vi "Schedule Packet Generation Based on Timestamps.vi"(0 "tagged llp packet":T1, 1 "reset":bool, 2 "generation counter":T10, 5 "start trigger":bool, 7 "stop trigger":bool, 9 "tagged llp packet valid":bool, 11 "configuration":T11, 12 "ready to generate packet":bool) -> (3 "in reset":bool, 4 "packet timing error":bool, 6 "packet timing error (cycles)":u64, 8 "number of buffered llp timestamps":u32, 10 "generate packet":bool, 14 "ready for tagged llp packet":bool)   [LabVIEW 2020, in "GettingStarted_Gen_148X_FPGA.lvlib"]
uses:
  GettingStarted_Gen_148X_FPGA.lvlib
  Types/Serial Output Channel Datapath Configuration.ctl
  <instrlib>/FlexRIO/CSI-2/v2/FPGA/Types/Timestamp Counter Value.ctl
  <instrlib>/FlexRIO/CSI-2/v2/FPGA/Types/Tagged LLP Packet.ctl
  <instrlib>/FlexRIO/CSI-2/v2/FPGA/Types/FPGA LLP Packet Tag.ctl
  <instrlib>/FlexRIO/CSI-2/v2/FPGA/Types/FPGA LLP Packet Timestamp.ctl
  <instrlib>/FlexRIO/CSI-2/v2/FPGA/Types/Timestamp ID.ctl
  <instrlib>/FlexRIO/CSI-2/v2/FPGA/Types/FPGA LLP Packet Size.ctl
  <instrlib>/FlexRIO/CSI-2/v2/FPGA/Types/LLP Packet.ctl
  <instrlib>/FlexRIO/CSI-2/v2/FPGA/Types/LLP Packet Header.ctl
  <instrlib>/FlexRIO/CSI-2/v2/FPGA/Types/LLP Packet Payload.ctl
  <instrlib>/FlexRIO/CSI-2/v2/FPGA/Types/LLP Packet Footer.ctl
  <instrlib>/FlexRIO/CSI-2/v2/FPGA/NI CSI-2 API FPGA v2.lvlib
  <instrlib>/_niInstr/Basic Elements/v1/FPGA/niInstr Basic Elements v1 FPGA.lvlib
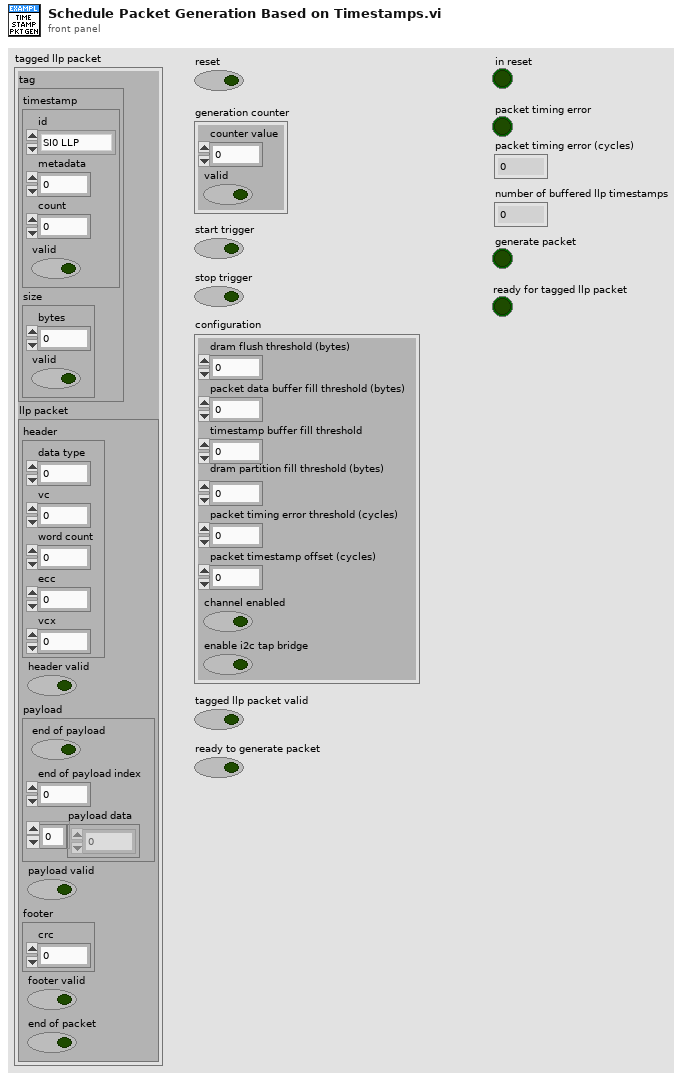
[diagram p1: front panel]
types:
  T1 = typedef "NI CSI-2 API FPGA v2.lvlib/Tagged LLP Packet.ctl" = cluster{"tag":T2, "llp packet":T6}
  T2 = typedef "NI CSI-2 API FPGA v2.lvlib/FPGA LLP Packet Tag.ctl" = cluster{"timestamp":T3, "size":T5}
  T3 = typedef "NI CSI-2 API FPGA v2.lvlib/FPGA LLP Packet Timestamp.ctl" = cluster{"valid":bool, "count":fxp<+,50,50>, "id":T4, "metadata":u8}
  T4 = typedef "NI CSI-2 API FPGA v2.lvlib/Timestamp ID.ctl" = enum8{"SI0 LLP", "SI1 LLP", "SI2 LLP", "SI3 LLP", "SI4 LLP", "SI5 LLP", "SI6 LLP", "SI7 LLP", "SO0 LLP", "SO1 LLP", "SO2 LLP", "SO3 LLP", "SO4 LLP", "SO5 LLP", "SO6 LLP", "SO7 LLP", "Ser0 GPIO Bank", "Ser1 GPIO Bank", "Ser2 GPIO Bank", "Ser3 GPIO Bank", "Ser4 GPIO Bank", "Ser5 GPIO Bank", "Ser6 GPIO Bank", "Ser7 GPIO Bank", "Des0 GPIO Bank", "Des1 GPIO Bank", "Des2 GPIO Bank", "Des3 GPIO Bank", "Des4 GPIO Bank", "Des5 GPIO Bank", "Des6 GPIO Bank", "Des7 GPIO Bank", "User0", "User1", "User2", "User3", "User4", "User5", "User6", "User7", "User8", "User9", "User10", "User11", "User12", "User13", "User14", "User15", "User16", "User17", "User18", "User19", "User20", "User21", "User22", "User23", "User24", "User25", "User26", "User27", "User28", "User29", "User30", "User31"}
  T5 = typedef "NI CSI-2 API FPGA v2.lvlib/FPGA LLP Packet Size.ctl" = cluster{"bytes":fxp<+,17,17>, "valid":bool}
  T6 = typedef "NI CSI-2 API FPGA v2.lvlib/LLP Packet.ctl" = cluster{"header":T7, "header valid":bool, "payload":T8, "payload valid":bool, "footer":T9, "footer valid":bool, "end of packet":bool}
  T7 = typedef "NI CSI-2 API FPGA v2.lvlib/LLP Packet Header.ctl" = cluster{"word count":u16, "ecc":fxp<+,6,6>, "vcx":fxp<+,2,2>, "data type":fxp<+,6,6>, "vc":fxp<+,2,2>}
  T8 = typedef "NI CSI-2 API FPGA v2.lvlib/LLP Packet Payload.ctl" = cluster{"end of payload":bool, "end of payload index":fxp<+,3,3>, "payload data":u8[]}
  T9 = typedef "NI CSI-2 API FPGA v2.lvlib/LLP Packet Footer.ctl" = cluster{"crc":u16}
  T10 = typedef "NI CSI-2 API FPGA v2.lvlib/Timestamp Counter Value.ctl" = cluster{"counter value":u64, "valid":bool}
  T11 = typedef "GettingStarted_Gen_148X_FPGA.lvlib/Serial Output Channel Datapath Configuration.ctl" = cluster{"dram flush threshold (bytes)":u64, "packet data buffer fill threshold (bytes)":u64, "timestamp buffer fill threshold":u32, "packet timing error threshold (cycles)":u64, "channel enabled":bool, "dram partition fill threshold (bytes)":u64, "enable i2c tap bridge":bool, "packet timestamp offset (cycles)":i64}
  T12 = typedef "NI CSI-2 API FPGA v2.lvlib/Raw Timestamp.ctl" = cluster{"timestamp":u64, "valid":bool}
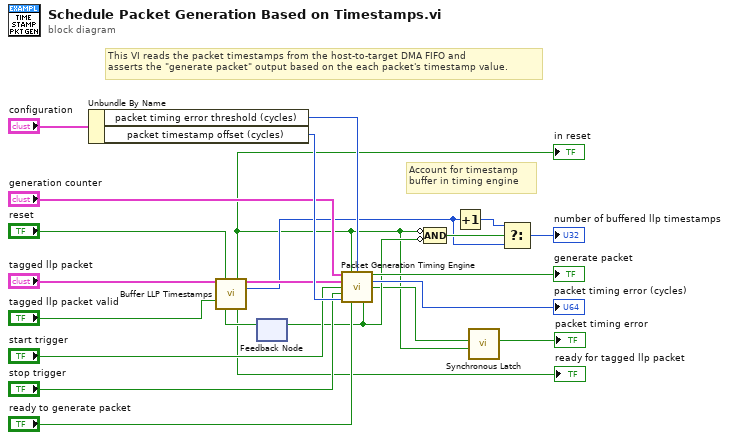
[diagram p0: block diagram]
diagram:
  # "Account for timestamp \nbuffer in timing engine"
  # "This VI reads the packet timestamps from the host-to-target DMA FIFO and \nasserts the \"generate packet\" output based on the each packet's timestamp value."
  n1 = Unbundle By Name("configuration") -> ("packet timing error threshold (cycles)"=w20:u64, "packet timestamp offset (cycles)"=w23:i64)
  n2 = feedback #1() -> (w17:bool)  [unwired: 1 in]
  n3 = call "Buffer LLP Timestamps.vi"("tagged llp packet"="tagged llp packet", "reset"="reset", "input valid"="tagged llp packet valid", "ready for ouput"=w17) -> ("in reset"=w1:bool, "llp timestamp"=w16:T12, "number of timestamps in fifo"=w8:u32, "ready for input"=→"ready for tagged llp packet":bool)  [unwired: 8 in]
  "in reset" <- w1
  n4 = call <instrlib>:"Packet Generation Timing Engine.vi"("counter value"="generation counter", "reset"=w1, "packet timing error threshold (cycles)"=w20, "packet timestamp"=w16, "start trigger"="start trigger", "stop trigger"="stop trigger", "packet timestamp offset (cycles)"=w23, "ready for output"="ready to generate packet") -> ("generate packet"=→"generate packet":bool, "packet timing error (cycles)"=→"packet timing error (cycles)":u64, "packet timing error"=w3:bool, "ready for packet timestamp"=w12:bool)  [unwired: 4 in]
  n5 = feedback-in #1(w12) -> ()
  n6 = Compound Arithmetic op=AND(invert w1, invert w12) -> (w11:bool)
  n7 = Increment(x=w8) -> (x+1=w10:u32)
  n8 = call <instrlib>:"Synchronous Latch.vi"("clear"=w1, "set"=w3) -> ("out"=→"packet timing error":bool)  [unwired: 9 in]
  n9 = Select(t=w10, s=w11, f=w8) -> (s? t:f=→"number of buffered llp timestamps":u32)
